vi "Default Instrument Setup.vi"(8 "error in (no error)":errorcluster, 11 "VISA resource name":refnum<visa-resource-name>) -> (0 "error out":errorcluster, 3 "VISA resource name out":refnum<visa-resource-name>)   [LabVIEW 2013, in "YbTempCtrl.lvlib"]
doc: "Sends a default command string to the instrument whenever a new VISA session is opened, or the instrument is reset. Use this VI as a subVI for the <b>Initialize</b> and <b>Reset</b> VIs. Altering this VI could cause these two VIs to operate incorrectly."
uses:
  YbTempCtrl.lvlib
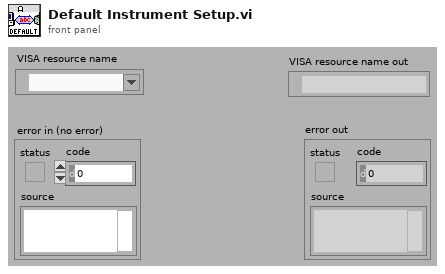
[diagram p1: front panel]
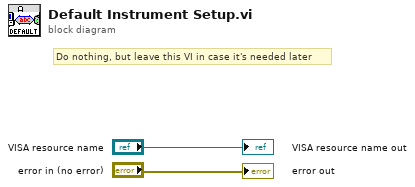
[diagram p0: block diagram]
diagram:
  # "Do nothing, but leave this VI in case it's needed later"
  "error out" <- "error in (no error)"
  "VISA resource name out" <- "VISA resource name"
